vi "FPGAController_v4.vi"() -> ()   [LabVIEW 2013]
uses:
  <vilib>/Utility/miscctls.llb/LVPointTypeDef.ctl
  <userlib>/_OpenG.lib/file/file.llb/Strip Path Extension - Path__ogtk.vi
  <userlib>/_OpenG.lib/comparison/comparison.llb/Boolean Changed__ogtk.vi
  <vilib>/FPGAPlugInAG/PXI-7954R/niLvFpga_Open_PXI-7954R.vi
  <vilib>/addons/database/Connection.llb/Conn Execute.vi
  <vilib>/addons/database/Recordset.llb/Rec Fetch Recordset Data (R).vi
  <vilib>/addons/database/Recordset.llb/Rec Destroy - Connection.vi
  <vilib>/Utility/error.llb/Error Cluster From Error Code.vi
  <vilib>/rvi/errors/niLvFpgaAdjustHostInterfaceError.vi
  <vilib>/FPGAPlugInAG/PXI-7954R/niLvFpga_Close_PXI-7954R.vi
  <vilib>/rvi/interface/nirviOpenFPGA/nirviOpenFPGA.xnode
  FPGA Bitfiles/correlationwithf_FPGATarget_FPGAcode60214_dpdmgs7o1BA.lvbitx
  <vilib>/rvi/interface/nirviMethod/nirviMethod.xnode
  <vilib>/FPGA/interface/niFpgaViExecutionMode.ctl
  <vilib>/rvi/interface/nirviReadWriteControl/nirviReadWriteControl.xnode
  <vilib>/addons/database/_DB Variant To Data/Database Variant To Data.xnode
  <vilib>/rvi/interface/nirviCloseFPGA/nirviCloseFPGA.xnode
  <vilib>/addons/database/NI_Database_API.lvlib
  NiFpgaLv.dll
panel:
  in  "Lower Threshold":bool
  in  "Raise Threshold":bool
  out "Update Threshold":bool
  in  "Min. Time\nBetween Shots (s)":dbl
  in  "Rate Limiting":bool
  out "Armed":bool
  in  "Use Delay?":bool
  in  "Add Delay":bool
  in  "Delay Name":string
  in  "Delay Value":dbl=3.0
  in  "Delay Ring":dbl(ring)=3.15039 items=["Ablation Chamber"=6.45, "LEIL Chamber"=4.318, "Thid Detector"=3.15039, "Custom"=0.0]
  in  "Rearm Trigger":bool
  in  "One Shot Mode":bool
  out "Last Update:":timestamp
  out "Updating FPGA":bool
  out "Sensitivity":dbl
  out "error out":errorcluster
  out "Low Mass Limit":fxp<+,31,17>
  out "High Mass Limit":fxp<+,31,17>
  out "stopping":bool
  in  "Auto Threshold":bool
  out "Peletron (MV)":dbl=2.0
  out "High Mass (kg)":dbl=inf
  out "Low Mass (kg)":dbl
  out "High Charge Limit":i16
  out "Low Charge Limit":i16
  out "High velocity count":i32=210
  out "Low velocity count":i32=21000
  in  "stop":bool
  in  "Peak-Threshold Factor":dbl=2.0
  out "Low Charge Limit (fC)":dbl
  out "High Charge Limit (fC)":dbl=100.0
  out "High Velocity":dbl=100000.0
  out "Low Velocity":dbl=1000.0
  out "Filter 7 Peak":i32=7483
  out "Filter 6 Peak":i32=9863
  out "Filter 5 Peak":i32=13910
  out "Filter 4 Peak":i32=18191
  out "Filter 3 Peak":i32=46254
  out "Filter 2 Peak":i32=120664
  out "Filter 1 Peak":i32=295996
  in  "Filter7 Threshold":i32=-21165
  in  "Filter6 Threshold":i32=-29358
  in  "Filter5 Threshold":i32=-41730
  in  "Filter4 Threshold":i32=-54306
  in  "Filter3 Threshold":i32=-138762
  in  "Filter2 Threshold":i32=-361992
  in  "Filter1 Threshold":i32=-887988
  in  "Zero Peak Values":bool
  in  "Assign Threshold":bool
  in  "Run Mode":bool
  # "Settings"
  # "Dubugging"
  # "Independent Variable"
  # "Low Vel."
  # "High Vel."
  # "Low Q (fC)"
  # "High Q (fC)"
  # "Plate Control While Loop Counter"
  # "Low Mass (kg)"
  # "High Mass (kg)"
  # "Sens. (V/pC)"
  # "Peletron (MV)"
  # "Current Value of Running Average"
  # "Peak Threshold Factor"
  # "Delay Trigger"
  # "Dist. from 2nd Det. (m)"
  # "Name"
  # "Peak Values"
  # "Peak 1"
  # "Peak 2"
  # "Peak 3"
  # "Peak 4"
  # "Peak 5"
  # "Peak 6"
  # "Peak 7"
  # "Thresholds"
  # "Threshold 1"
  # "Threshold 2"
  # "Threshold 3"
  # "Threshold 4"
  # "Threshold 5"
  # "Threshold 6"
  # "Threshold 7"
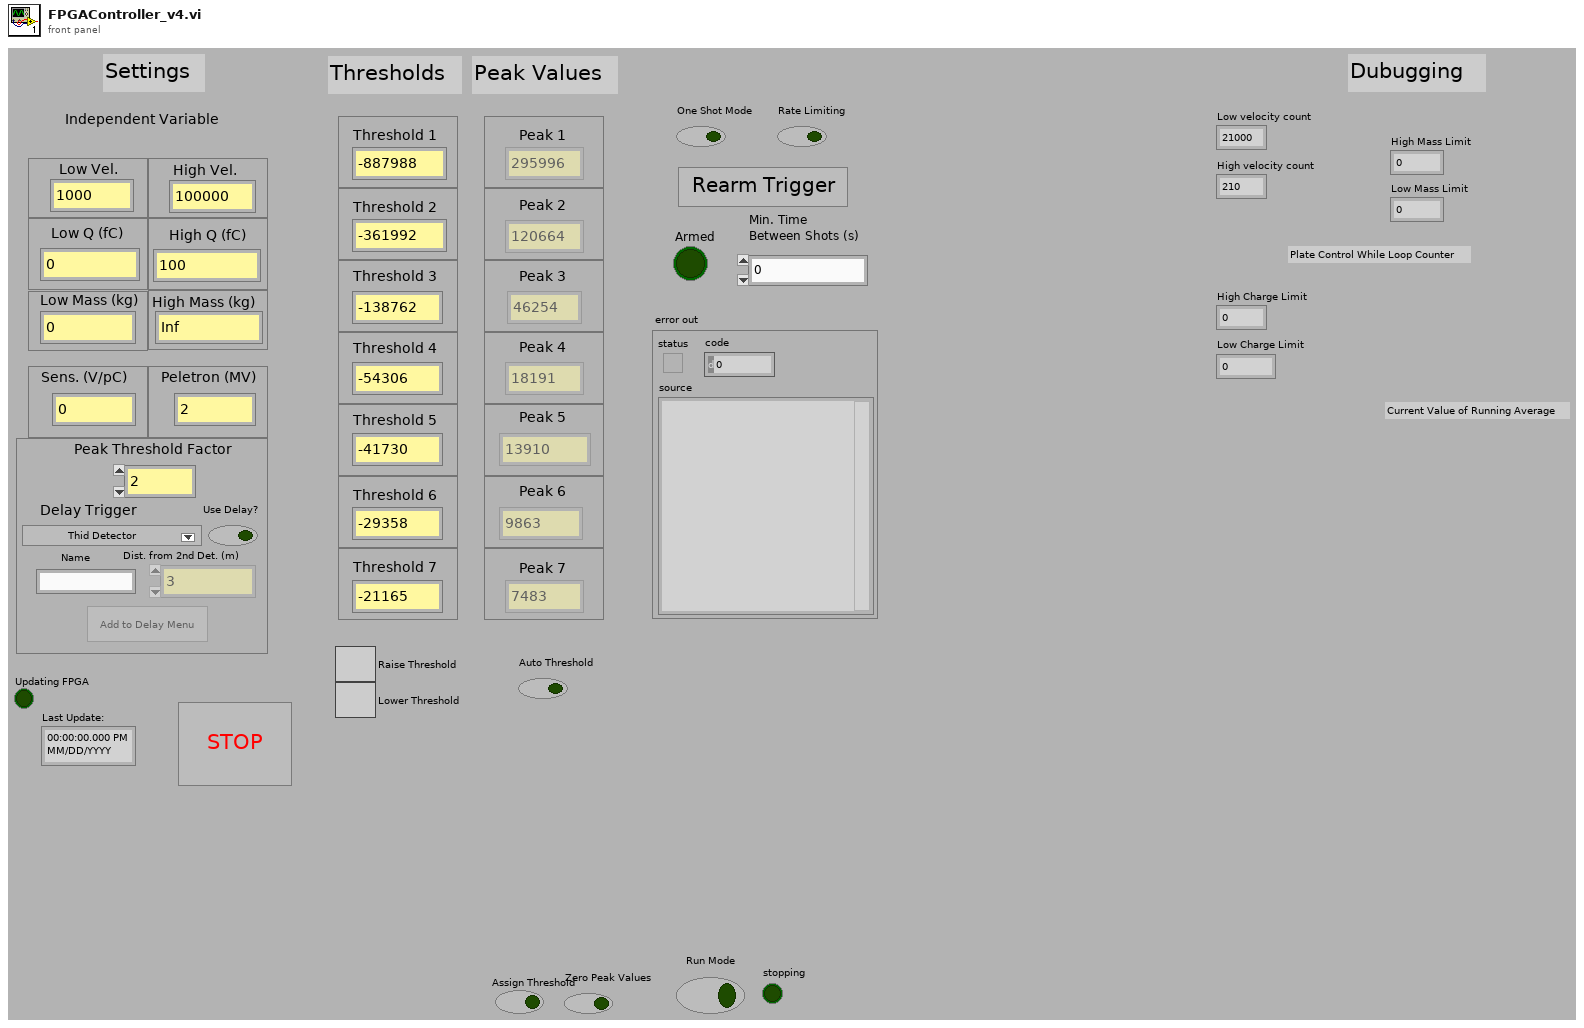
[diagram p1: front panel]
types:
  T1 = typedef "LVPointTypeDef.ctl" = cluster{"Horizontal":i16, "Vertical":i16}
  T2 = enum8{"Enabled", "Disabled", "Disabled and Grayed Out"}
  T3 = typedef "NI_Database_API.lvlib/Conn ObjectReference.ctl" = refnum<k1>
  T4 = cluster{"Filter 1 Peak":i32, "Filter 2 Peak":i32, "Filter 3 Peak":i32, "Filter 4 Peak":i32, "Filter 5 Peak":i32, "Filter 6 Peak":i32, "Filter 7 Peak":i32}
  T5 = typedef "NI_Database_API.lvlib/Rec ObjectReference.ctl" = refnum<k1>
  T6 = typedef "LVStringsAndValuesArrayTypeDef_DBL.ctl" = cluster{"String":string, "Value":dbl}[]
  T7 = cluster{"Numeric":dbl, "Numeric":dbl, "Numeric":dbl, "Numeric":dbl, "Numeric":dbl, "Numeric":dbl, dbl, dbl, "Value":dbl, fxp<+,16,7>, "Use Delay?":bool}
  T8 = cluster{"Low Velocity Count":i32, "High Velocity Count":i32, "Low Charge Limit (ADC ticks)":i16, "High Charge Limit (ADC ticks)":i16, "Low Mass (ADC*cycle^2)":i64, "High Mass (ADC*cycle^2)":i64, "Mult":fxp<+,16,7>, "Mult Use?":bool}
  T9 = cluster{"Filter 1 Detector 3 Correlation":i32, "Filter 2 Detector 3 Correlation":i32, "Filter 3 Detector 3 Correlation":i32, "Filter 4 Detector 3 Correlation":i32, "Filter 5 Detector 3 Correlation":i32, "Filter 6 Detector 3 Correlation":i32, "Filter 7 Detector 3 Correlation":i32}
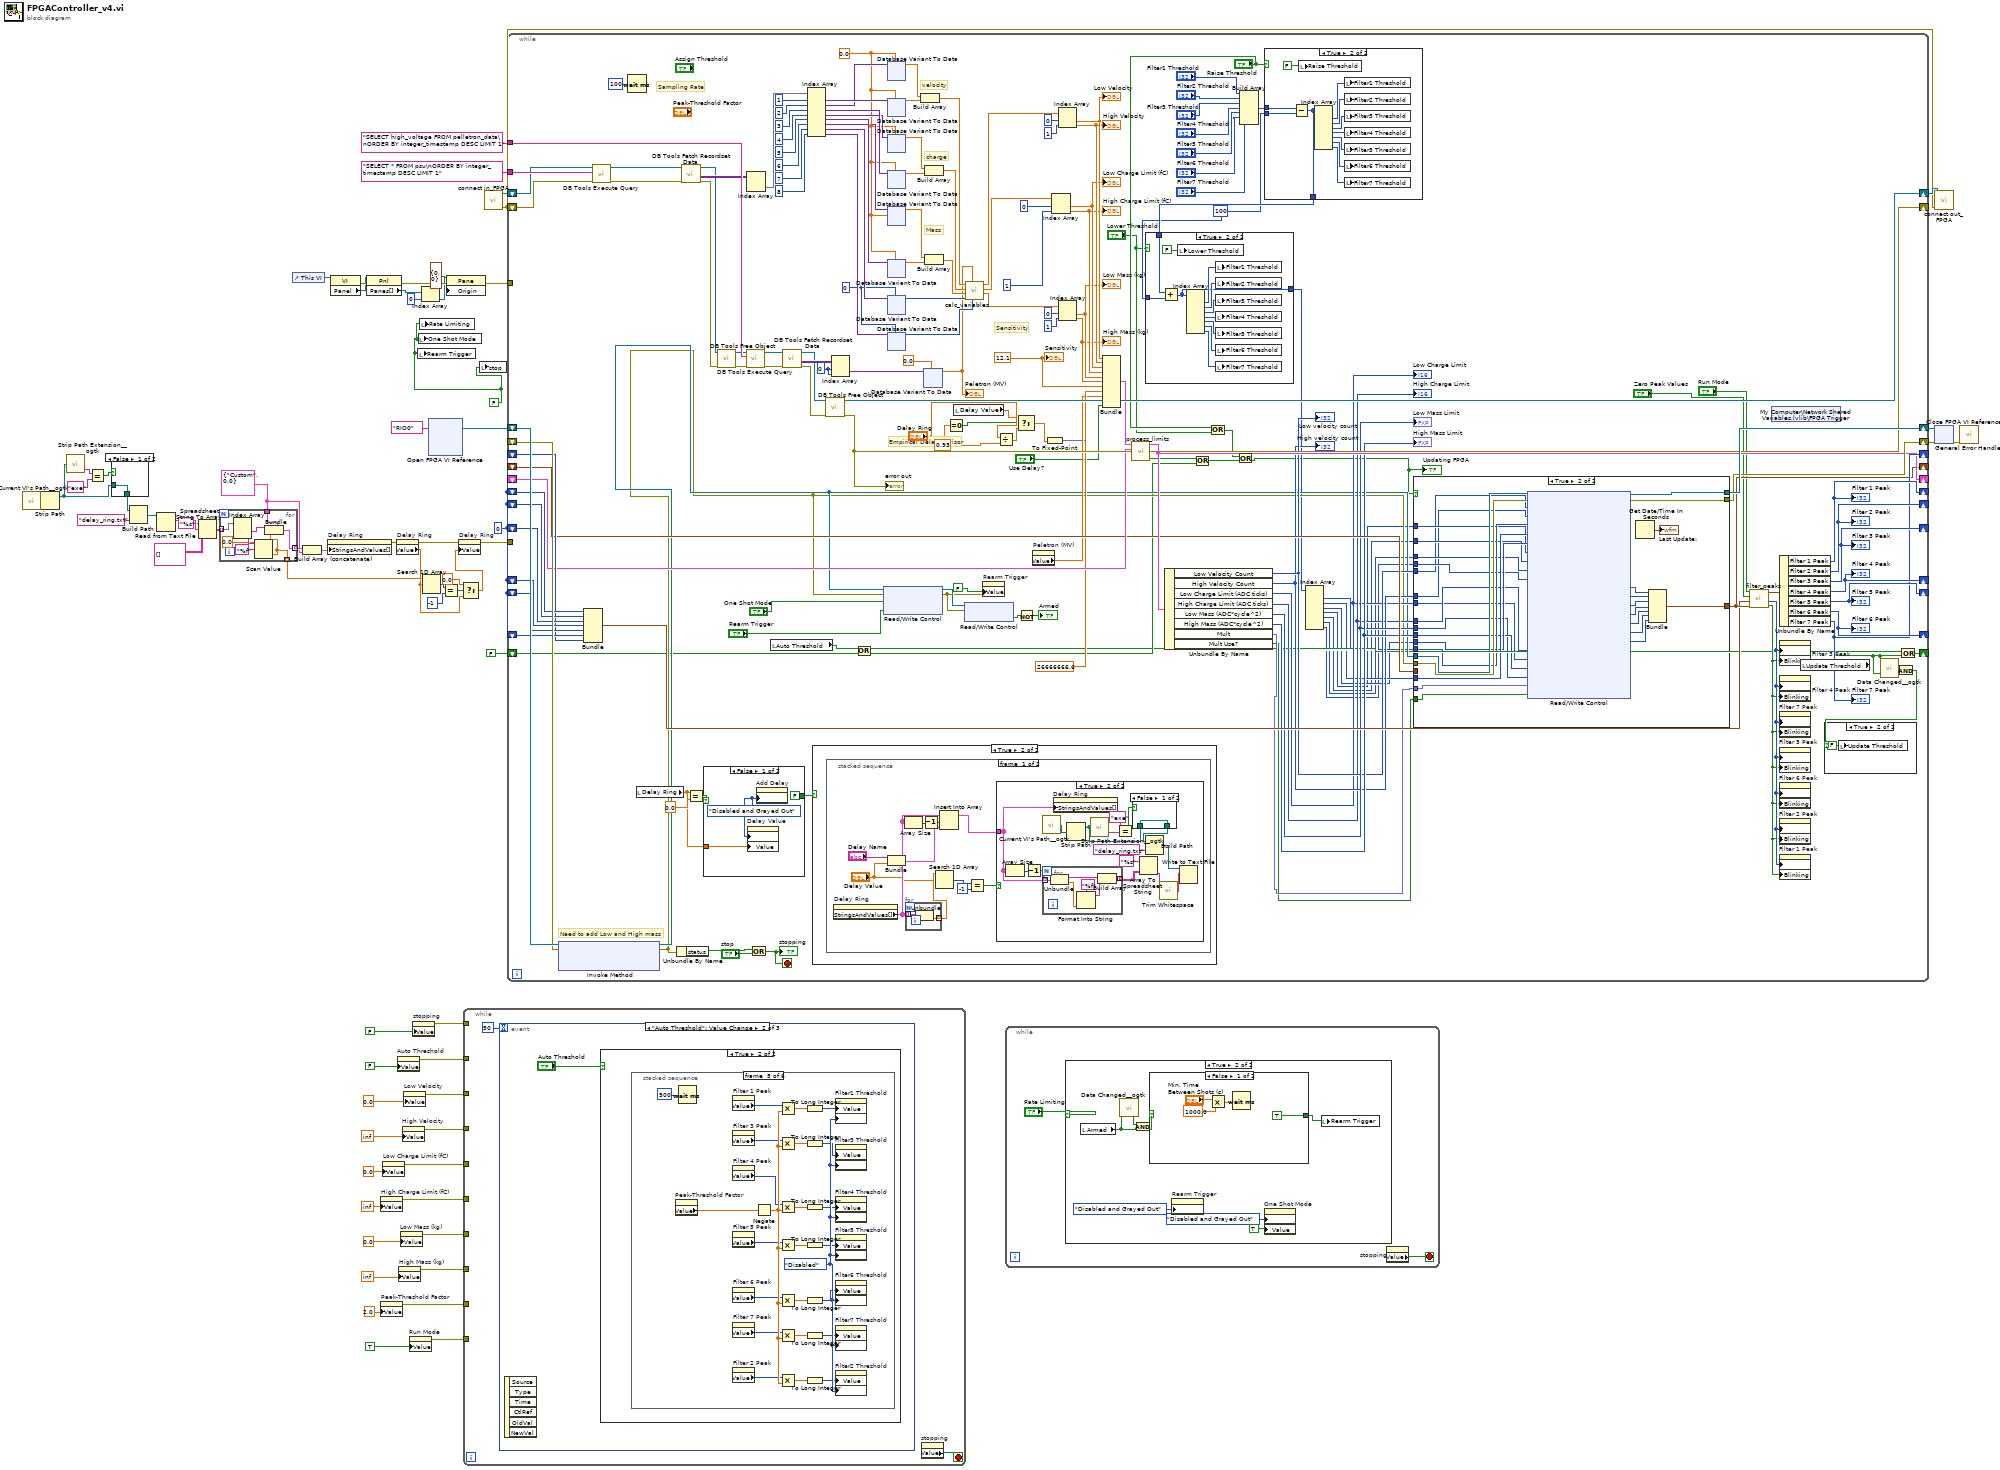
[diagram p0: block diagram]
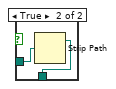
[diagram p2: hidden frame]
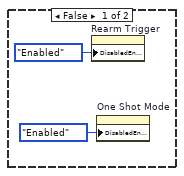
[diagram p3: hidden frame]
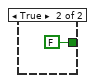
[diagram p4: hidden frame]
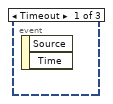
[diagram p5: hidden frame]
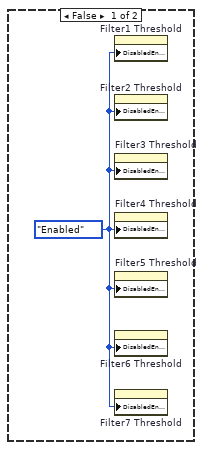
[diagram p6: hidden frame]
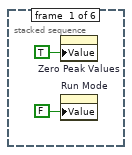
[diagram p7: hidden frame]
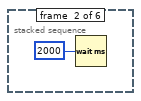
[diagram p8: hidden frame]
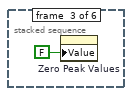
[diagram p9: hidden frame]
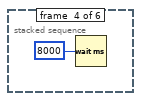
[diagram p10: hidden frame]
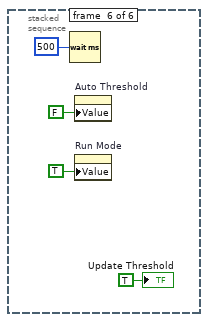
[diagram p11: hidden frame]
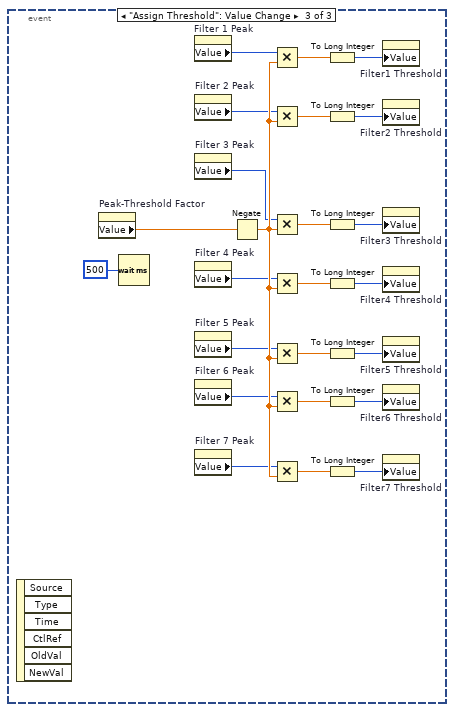
[diagram p12: hidden frame]
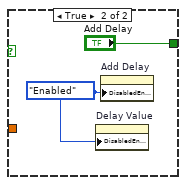
[diagram p16: hidden frame]
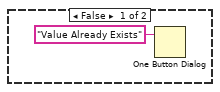
[diagram p18: hidden frame]
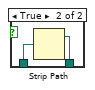
[diagram p19: hidden frame]
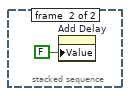
[diagram p20: hidden frame]
diagram:
  w17 = cluster{"String":string, "Value":dbl} {"String"="Custom", "Value"=0.0}
  w27 = FALSE
  w66 = 0
  n1 = call <userlib>:"Current VI's Path__ogtk.vi"() -> ("Current VI's Path (+ Relative)"=w26:path)  [unwired: 1 in]
  n2 = Strip Path(path=w26) -> (stripped path=w12:path)  [unwired: 1 out]
  n3 = call-poly <userlib>:"Strip Path Extension__ogtk.vi"("path"=w12) -> ("extension"=w16:string)  [unwired: 1 out]
  n4 = Equal?(x=w16, y="exe") -> (x = y?=w13:bool)
  n5 = case shown="False" w13 {
    tunnel: w12 -> [w68 w70]
    tunnel: [w68 w69] -> w11
    frame False {
    }
    frame True {
      n6 = Strip Path(path=w70) -> (stripped path=w69:path)  [unwired: 1 out]
    }
  }
  n7 = Build Path(base path=w11, name or relative path="delay_ring.txt") -> (appended path=w14:path)
  n8 = Read from Text File(file (use dialog)=w14) -> (text=w24:string)  [unwired: 3 in, 3 out]
  n9 = Spreadsheet String To Array(format string="%s", spreadsheet string=w24, array type (2D Dbl)=string[][] []) -> (array=w21:string[][])  [unwired: 1 in]
  n10 = for {
    tunnel: w21 -> [w78] mode=indexing
    tunnel: w17 -> [w76]
    tunnel: [w72] -> w18 mode=indexing
    tunnel: [w71] -> w10 mode=indexing
    n11 = Index Array(array=w78) -> (element #1=w77:string, element #2=w75:string)  [unwired: 2 in]
    n12 = Scan Value(string=w75, format string="%f", default (0 dbl)=0.0) -> (value=w71:dbl)  [unwired: 1 out]
    n13 = Bundle(cluster=w76, "String"=w77, "Value"=w71) -> (w72:cluster{"String":string, "Value":dbl})
  }
  n14 = control-ref of="This VI"() -> (w38:refnum<vi>)
  n15 = Build Array (concatenate)(w18, w17) -> (w20:cluster{"String":string, "Value":dbl}[])
  n16 = property on="Delay Ring" class="Ring (strict)"("StringsAndValues[]"=w20) -> (error out=w19:errorcluster)  [unwired: 2 in, 1 out]
  n17 = property class="VI"(reference=w38) -> (error out=w37:errorcluster, "Panel"=w36:refnum<vi>)  [unwired: 1 in, 1 out]
  n18 = property class="Pnl"(reference=w36, error in=w37) -> (error out=w35:errorcluster, "Panes[]"=w34:refnum<vi>[])  [unwired: 1 out]
  n19 = property on="High Charge Limit (fC)" class="DigNum (strict)"("Value"=inf ("High Charge Limit (fC)")) -> (error out=w53:errorcluster)  [unwired: 2 in, 1 out]
  n20 = property on="Peak-Threshold Factor" class="DigNum (strict)"("Value"=2.0 ("Peak-Threshold Factor")) -> (error out=w47:errorcluster)  [unwired: 2 in, 1 out]
  n21 = property on="Low Charge Limit (fC)" class="DigNum (strict)"("Value"=0.0 ("Low Charge Limit (fC)")) -> (error out=w55:errorcluster)  [unwired: 2 in, 1 out]
  n22 = property on="Delay Ring" class="Ring (strict)"(error in=w19) -> (error out=w9:errorcluster, "Value"=w3:dbl)  [unwired: 1 in, 1 out]
  n23 = property on="Auto Threshold" class="Bool (strict)"("Value"=FALSE ("Auto Threshold")) -> (error out=w61:errorcluster)  [unwired: 2 in, 1 out]
  n24 = property on="High Mass (kg)" class="DigNum (strict)"("Value"=inf ("High Mass (kg)")) -> (error out=w49:errorcluster)  [unwired: 2 in, 1 out]
  n25 = property on="Low Mass (kg)" class="DigNum (strict)"("Value"=0.0 ("Low Mass (kg)")) -> (error out=w51:errorcluster)  [unwired: 2 in, 1 out]
  n26 = property on="High Velocity" class="DigNum (strict)"("Value"=inf ("High Velocity")) -> (error out=w57:errorcluster)  [unwired: 2 in, 1 out]
  n27 = property on="Low Velocity" class="DigNum (strict)"("Value"=0.0 ("Low Velocity")) -> (error out=w59:errorcluster)  [unwired: 2 in, 1 out]
  n28 = property on="Run Mode" class="Bool (strict)"("Value"=TRUE ("Run Mode")) -> (error out=w45:errorcluster)  [unwired: 2 in, 1 out]
  n29 = property on="stopping" class="Bool (strict)"("Value"=FALSE ("stopping")) -> (error out=w63:errorcluster)  [unwired: 2 in, 1 out]
  n30 = local write "Rearm Trigger"(w27) -> ()
  n31 = local write "One Shot Mode"(w27) -> ()
  n32 = local write "Rate Limiting"(w27) -> ()
  n33 = Index Array(array=w34, index=0) -> (element=w32:refnum<vi>)
  n34 = Search 1D Array(1D array=w10, element=w3) -> (index of element=w7:i32)  [unwired: 1 in]
  n35 = xnode "Open FPGA VI Reference"("resource name"=tag "RIO0") -> ("FPGA VI Reference Out"=w29:refnum<k20>)  [unwired: 1 in, 1 out]
  n36 = Equal?(x=w7, y=-1) -> (x = y?=w5:bool)
  n37 = property class="Pane"(reference=w32, error in=w35, "Origin"=T1 {"Horizontal"=0, "Vertical"=0}) -> (error out=w30:errorcluster)  [unwired: 1 out]
  n38 = Select(t=0.0, s=w5, f=w3) -> (s? t:f=w4:dbl)
  n39 = property on="Delay Ring" class="Ring (strict)"(error in=w9, "Value"=w4) -> (error out=w8:errorcluster)  [unwired: 1 in, 1 out]
  n40 = while {
    tunnel: w63 -> [_]
    tunnel: w61 -> [_]
    tunnel: w59 -> [_]
    tunnel: w57 -> [_]
    tunnel: w55 -> [_]
    tunnel: w53 -> [_]
    tunnel: w51 -> [_]
    tunnel: w49 -> [_]
    tunnel: w47 -> [_]
    tunnel: w45 -> [_]
    stop <- w80 stop-if-true
    n41 = event shown="[1] \"Auto Threshold\": Value Change" {
      selector: _ -> [_ _ _]
      dyn-events: _ -> [_ _ _]
      timeout: 50 -> [_ _ _]
      event Timeout {
        n42 = event-data() -> ()  [unwired: 1 in, 2 out]
      }
      event "Auto Threshold": Value Change {
        n43 = event-data() -> ()  [unwired: 1 in, 6 out]
        n44 = case shown="True" "Auto Threshold" {
          frame False {
            w82 = T2."Enabled" ("Disabled")
            n45 = property on="Filter1 Threshold" class="DigNum (strict)"("DisabledEnum"=w82) -> ()  [unwired: 2 in, 2 out]
            n46 = property on="Filter2 Threshold" class="DigNum (strict)"("DisabledEnum"=w82) -> ()  [unwired: 2 in, 2 out]
            n47 = property on="Filter3 Threshold" class="DigNum (strict)"("DisabledEnum"=w82) -> ()  [unwired: 2 in, 2 out]
            n48 = property on="Filter4 Threshold" class="DigNum (strict)"("DisabledEnum"=w82) -> ()  [unwired: 2 in, 2 out]
            n49 = property on="Filter5 Threshold" class="DigNum (strict)"("DisabledEnum"=w82) -> ()  [unwired: 2 in, 2 out]
            n50 = property on="Filter6 Threshold" class="DigNum (strict)"("DisabledEnum"=w82) -> ()  [unwired: 2 in, 2 out]
            n51 = property on="Filter7 Threshold" class="DigNum (strict)"("DisabledEnum"=w82) -> ()  [unwired: 2 in, 2 out]
          }
          frame True {
            n52 = stacked-sequence {
              frame #0 {
                n53 = property on="Zero Peak Values" class="Bool (strict)"("Value"=TRUE ("Zero Peak Values")) -> ()  [unwired: 2 in, 2 out]
                n54 = property on="Run Mode" class="Bool (strict)"("Value"=FALSE ("Run Mode")) -> ()  [unwired: 2 in, 2 out]
              }
              frame #1 {
                n55 = Wait (ms)(milliseconds to wait=u32 2000) -> ()  [unwired: 1 out]
              }
              frame #2 {
                n56 = property on="Zero Peak Values" class="Bool (strict)"("Value"=FALSE ("Zero Peak Values")) -> ()  [unwired: 2 in, 2 out]
              }
              frame #3 {
                n57 = Wait (ms)(milliseconds to wait=u32 8000) -> ()  [unwired: 1 out]
              }
              frame #4 {
                w112 = T2."Disabled" ("Disabled")
                n58 = property on="Peak-Threshold Factor" class="DigNum (strict)"() -> ("Value"=w97:dbl)  [unwired: 2 in, 2 out]
                n59 = Wait (ms)(milliseconds to wait=u32 500) -> ()  [unwired: 1 out]
                n60 = property on="Filter 1 Peak" class="DigNum (strict)"() -> ("Value"=w95:i32)  [unwired: 2 in, 2 out]
                n61 = property on="Filter 3 Peak" class="DigNum (strict)"() -> ("Value"=w93:i32)  [unwired: 2 in, 2 out]
                n62 = property on="Filter 4 Peak" class="DigNum (strict)"() -> ("Value"=w92:i32)  [unwired: 2 in, 2 out]
                n63 = property on="Filter 5 Peak" class="DigNum (strict)"() -> ("Value"=w91:i32)  [unwired: 2 in, 2 out]
                n64 = property on="Filter 6 Peak" class="DigNum (strict)"() -> ("Value"=w90:i32)  [unwired: 2 in, 2 out]
                n65 = property on="Filter 7 Peak" class="DigNum (strict)"() -> ("Value"=w89:i32)  [unwired: 2 in, 2 out]
                n66 = property on="Filter 2 Peak" class="DigNum (strict)"() -> ("Value"=w94:i32)  [unwired: 2 in, 2 out]
                n67 = Negate(x=w97) -> (-x=w96:dbl)
                n68 = Multiply(x=w95, y=w96) -> (x*y=w111:dbl)
                n69 = Multiply(x=w93, y=w96) -> (x*y=w107:dbl)
                n70 = Multiply(x=w92, y=w96) -> (x*y=w105:dbl)
                n71 = Multiply(x=w91, y=w96) -> (x*y=w103:dbl)
                n72 = Multiply(x=w90, y=w96) -> (x*y=w101:dbl)
                n73 = Multiply(x=w89, y=w96) -> (x*y=w99:dbl)
                n74 = Multiply(x=w94, y=w96) -> (x*y=w109:dbl)
                n75 = To Long Integer(number=w111) -> (32bit integer=w110:i32)
                n76 = To Long Integer(number=w107) -> (32bit integer=w106:i32)
                n77 = To Long Integer(number=w105) -> (32bit integer=w104:i32)
                n78 = To Long Integer(number=w103) -> (32bit integer=w102:i32)
                n79 = To Long Integer(number=w101) -> (32bit integer=w100:i32)
                n80 = To Long Integer(number=w99) -> (32bit integer=w98:i32)
                n81 = To Long Integer(number=w109) -> (32bit integer=w108:i32)
                n82 = property on="Filter1 Threshold" class="DigNum (strict)"("Value"=w110, "DisabledEnum"=w112) -> ()  [unwired: 2 in, 2 out]
                n83 = property on="Filter3 Threshold" class="DigNum (strict)"("Value"=w106, "DisabledEnum"=w112) -> ()  [unwired: 2 in, 2 out]
                n84 = property on="Filter4 Threshold" class="DigNum (strict)"("Value"=w104, "DisabledEnum"=w112) -> ()  [unwired: 2 in, 2 out]
                n85 = property on="Filter5 Threshold" class="DigNum (strict)"("Value"=w102, "DisabledEnum"=w112) -> ()  [unwired: 2 in, 2 out]
                n86 = property on="Filter6 Threshold" class="DigNum (strict)"("Value"=w100, "DisabledEnum"=w112) -> ()  [unwired: 2 in, 2 out]
                n87 = property on="Filter7 Threshold" class="DigNum (strict)"("Value"=w98, "DisabledEnum"=w112) -> ()  [unwired: 2 in, 2 out]
                n88 = property on="Filter2 Threshold" class="DigNum (strict)"("Value"=w108, "DisabledEnum"=w112) -> ()  [unwired: 2 in, 2 out]
              }
              frame #5 {
                n89 = Wait (ms)(milliseconds to wait=u32 500) -> ()  [unwired: 1 out]
                n90 = property on="Auto Threshold" class="Bool (strict)"("Value"=FALSE ("Auto Threshold")) -> ()  [unwired: 2 in, 2 out]
                n91 = property on="Run Mode" class="Bool (strict)"("Value"=TRUE ("Run Mode")) -> ()  [unwired: 2 in, 2 out]
                "Update Threshold" <- TRUE ("Update Threshold")
              }
            }
          }
        }
      }
      event "Assign Threshold": Value Change {
        n92 = event-data() -> ()  [unwired: 1 in, 6 out]
        n93 = property on="Peak-Threshold Factor" class="DigNum (strict)"() -> ("Value"=w131:dbl)  [unwired: 2 in, 2 out]
        n94 = Wait (ms)(milliseconds to wait=u32 500) -> ()  [unwired: 1 out]
        n95 = property on="Filter 1 Peak" class="DigNum (strict)"() -> ("Value"=w130:i32)  [unwired: 2 in, 2 out]
        n96 = property on="Filter 2 Peak" class="DigNum (strict)"() -> ("Value"=w129:i32)  [unwired: 2 in, 2 out]
        n97 = property on="Filter 3 Peak" class="DigNum (strict)"() -> ("Value"=w128:i32)  [unwired: 2 in, 2 out]
        n98 = property on="Filter 4 Peak" class="DigNum (strict)"() -> ("Value"=w127:i32)  [unwired: 2 in, 2 out]
        n99 = property on="Filter 5 Peak" class="DigNum (strict)"() -> ("Value"=w126:i32)  [unwired: 2 in, 2 out]
        n100 = property on="Filter 6 Peak" class="DigNum (strict)"() -> ("Value"=w125:i32)  [unwired: 2 in, 2 out]
        n101 = property on="Filter 7 Peak" class="DigNum (strict)"() -> ("Value"=w124:i32)  [unwired: 2 in, 2 out]
        n102 = Negate(x=w131) -> (-x=w133:dbl)
        n103 = Multiply(x=w130, y=w133) -> (x*y=w140:dbl)
        n104 = Multiply(x=w129, y=w133) -> (x*y=w138:dbl)
        n105 = Multiply(x=w128, y=w133) -> (x*y=w137:dbl)
        n106 = Multiply(x=w127, y=w133) -> (x*y=w136:dbl)
        n107 = Multiply(x=w126, y=w133) -> (x*y=w135:dbl)
        n108 = Multiply(x=w125, y=w133) -> (x*y=w134:dbl)
        n109 = Multiply(x=w124, y=w133) -> (x*y=w139:dbl)
        n110 = To Long Integer(number=w140) -> (32bit integer=w123:i32)
        n111 = To Long Integer(number=w138) -> (32bit integer=w122:i32)
        n112 = To Long Integer(number=w137) -> (32bit integer=w121:i32)
        n113 = To Long Integer(number=w136) -> (32bit integer=w120:i32)
        n114 = To Long Integer(number=w135) -> (32bit integer=w119:i32)
        n115 = To Long Integer(number=w134) -> (32bit integer=w118:i32)
        n116 = To Long Integer(number=w139) -> (32bit integer=w117:i32)
        n117 = property on="Filter1 Threshold" class="DigNum (strict)"("Value"=w123) -> ()  [unwired: 2 in, 2 out]
        n118 = property on="Filter2 Threshold" class="DigNum (strict)"("Value"=w122) -> ()  [unwired: 2 in, 2 out]
        n119 = property on="Filter3 Threshold" class="DigNum (strict)"("Value"=w121) -> ()  [unwired: 2 in, 2 out]
        n120 = property on="Filter4 Threshold" class="DigNum (strict)"("Value"=w120) -> ()  [unwired: 2 in, 2 out]
        n121 = property on="Filter5 Threshold" class="DigNum (strict)"("Value"=w119) -> ()  [unwired: 2 in, 2 out]
        n122 = property on="Filter6 Threshold" class="DigNum (strict)"("Value"=w118) -> ()  [unwired: 2 in, 2 out]
        n123 = property on="Filter7 Threshold" class="DigNum (strict)"("Value"=w117) -> ()  [unwired: 2 in, 2 out]
      }
    }
    n124 = property on="stopping" class="Bool (strict)"() -> ("Value"=w80:bool)  [unwired: 2 in, 2 out]
  }
  n125 = local write "stop"(w27) -> ()
  n126 = call "connect in_FPGA.vi"() -> ("error out"=w39:errorcluster, "Database Connection"=w40:T3)  [unwired: 7 in, 1 out]
  n127 = while {
    shift-right: [w299] -> w65
    shift-left: w29 -> [w303]
    shift-right: [w298] -> w64
    shift-left: _ -> [w302]
    shift-right: [w294] -> _
    shift-left: w66 -> [w287]
    shift-right: [w293] -> _
    shift-left: w66 -> [w286]
    shift-right: [w292] -> _
    shift-left: w66 -> [w285]
    shift-right: [w291] -> _
    shift-left: w66 -> [w284]
    shift-right: [w290] -> _
    shift-left: w66 -> [w283]
    shift-right: [w296] -> _
    shift-left: w66 -> [w289]
    shift-right: [w295] -> _
    shift-left: w66 -> [w288]
    tunnel: "SELECT * FROM psu\nORDER BY integer_timestamp DESC LIMIT 1" ("SQL query") -> [w282]
    tunnel: "SELECT high_voltage FROM pelletron_data\nORDER BY integer_timestamp DESC LIMIT 1" ("SQL query") -> [w281]
    shift-right: [w277] -> w41
    shift-left: w40 -> [w280]
    shift-right: [w278] -> _
    shift-left: w39 -> [w279]
    shift-right: [w276] -> _
    shift-left: _ -> [w275]
    shift-right: [w273] -> _
    shift-left: _ -> [w274]
    tunnel: w30 -> [_]
    tunnel: w8 -> [_]
    shift-right: [w173] -> _
    shift-left: FALSE -> [w176]
    stop <- w297 stop-if-true
    w167 = 100
    w229 = 0 ("index (row)")
    w237 = i8 0
    w238 = 0.0
    w203 = 12.1
    # "charge"
    # "Empirical Delay Divisor"
    # "Mass"
    # "velocity"
    # "Sensitivity"
    # "Sampling Rate"
    # "Need to add Low and High mass"
    n128 = xnode "Invoke Method"("FPGA VI Reference In"=w303, "error in"=w302) -> ("FPGA VI Reference Out"=w196:refnum<k20>, "error out"=w195:errorcluster)  [unwired: 1 out]
    n129 = Bundle("Filter 1 Peak"=w289, "Filter 2 Peak"=w288, "Filter 3 Peak"=w287, "Filter 4 Peak"=w286, "Filter 5 Peak"=w285, "Filter 6 Peak"=w284, "Filter 7 Peak"=w283) -> (w269:T4)  [unwired: 1 in]
    n130 = call-poly <vilib>:"DB Tools Execute Query.vi"("error in (no error)"=w279, "SQL query"=w282, "connection reference"=w280) -> ("error out"=w257:errorcluster, "recordset reference"=w258:T5)  [unwired: 5 in]
    n131 = Wait (ms)(milliseconds to wait=u32 100) -> ()  [unwired: 1 out]
    n132 = local read "Delay Ring"() -> (w177:dbl)
    n133 = Unbundle By Name(w195) -> ("status"=w301:bool)
    n134 = call-poly <vilib>:"DB Tools Fetch Recordset Data.vi"("error in (no error)"=w257, "recordset reference"=w258) -> ("error out"=w235:errorcluster, "recordset data"=w248:variant[][], "recordset reference out"=w236:T5)  [unwired: 3 in]
    n135 = Equal?(x=w177, y=0.0) -> (x = y?=w178:bool)
    n136 = case shown="False" w178 {
      tunnel: [FALSE ("Add Delay") "Add Delay"] -> w200
      tunnel: w177 -> [w330 _]
      frame False {
        w331 = T2."Disabled and Grayed Out" ("Disabled")
        n137 = property on="Delay Value" class="DigNum (strict)"("DisabledEnum"=w331, "Value"=w330) -> ()  [unwired: 2 in, 2 out]
        n138 = property on="Add Delay" class="Bool (strict)"("DisabledEnum"=w331) -> ()  [unwired: 2 in, 2 out]
      }
      frame True {
        w332 = T2."Enabled" ("Disabled")
        n139 = property on="Delay Value" class="DigNum (strict)"("DisabledEnum"=w332) -> ()  [unwired: 2 in, 2 out]
        n140 = property on="Add Delay" class="Bool (strict)"("DisabledEnum"=w332) -> ()  [unwired: 2 in, 2 out]
      }
    }
    n141 = call-poly <vilib>:"DB Tools Free Object.vi"("error in (no error)"=w235, "recordset reference"=w236) -> ("error out"=w233:errorcluster, "connection reference"=w234:T3)  [unwired: 8 in]
    n142 = call-poly <vilib>:"DB Tools Execute Query.vi"("error in (no error)"=w233, "SQL query"=w281, "connection reference"=w234) -> ("error out"=w231:errorcluster, "recordset reference"=w232:T5)  [unwired: 5 in]
    n143 = Index Array(array=w248) -> (element=w247:variant[])  [unwired: 2 in]
    n144 = Or(x=w301, y="stop") -> (x .or. y?=w297:bool)
    "stopping" <- w297
    n145 = local read "Auto Threshold"() -> (w174:bool)
    n146 = call-poly <vilib>:"DB Tools Fetch Recordset Data.vi"("error in (no error)"=w231, "recordset reference"=w232) -> ("error out"=w204:errorcluster, "recordset data"=w230:variant[][], "recordset reference out"=w205:T5)  [unwired: 3 in]
    n147 = Index Array(array=w247, index #1=1 ("index"), index #2=2 ("index"), index #3=3 ("index"), index #4=4 ("index"), index #5=5 ("index"), index #6=6 ("index"), index #7=7 ("index"), index #8=8 ("index")) -> (element #1=w246:variant, element #2=w245:variant, element #3=w244:variant, element #4=w243:variant, element #5=w242:variant, element #6=w241:variant, element #7=w240:variant, element #8=w239:variant)
    n148 = case shown="True" w200 {
      frame False {
      }
      frame True {
        n149 = stacked-sequence {
          frame #0 {
            n150 = property on="Delay Ring" class="Ring (strict)"() -> ("StringsAndValues[]"=w336:T6)  [unwired: 2 in, 2 out]
            n151 = Bundle("Delay Name"="Delay Name", "Delay Value"="Delay Value") -> (w341:cluster{"Delay Name":string, "Delay Value":dbl})  [unwired: 1 in]
            n152 = Array Size(array=w336) -> (size(s)=w339:i32)
            n153 = for {
              tunnel: w336 -> [w346] mode=indexing
              tunnel: [w345] -> w335 mode=indexing
              n154 = Unbundle(w346) -> ("Value"=w345:dbl)  [unwired: 1 out]
            }
            n155 = Decrement(x=w339) -> (x-1=w338:i32)
            n156 = Search 1D Array(1D array=w335, element="Delay Value") -> (index of element=w343:i32)  [unwired: 1 in]
            n157 = Insert Into Array(array=w336, index=w338, new element=w341) -> (w340:T6)
            n158 = Equal?(x=w343, y=-1) -> (x = y?=w337:bool)
            n159 = case shown="True" w337 {
              tunnel: w340 -> [_ w355]
              frame False {
                n160 = One Button Dialog(message="Value Already Exists") -> ()  [unwired: 1 in, 1 out]
              }
              frame True {
                n161 = Array Size(array=w355) -> (size(s)=w357:i32)
                n162 = Decrement(x=w357) -> (x-1=w356:i32)
                n163 = call <userlib>:"Current VI's Path__ogtk.vi"() -> ("Current VI's Path (+ Relative)"=w361:path)  [unwired: 1 in]
                n164 = for {
                  N: w356 -> [_]
                  tunnel: w355 -> [w371] mode=indexing
                  tunnel: [w366] -> w358 mode=indexing
                  n165 = Unbundle(w371) -> ("String"=w367:string, "Value"=w370:dbl)
                  n166 = Format Into String(format string="%f", w370) -> (resulting string=w368:string)  [unwired: 2 in, 1 out]
                  n167 = Build Array(w367, w368) -> (w366:string[])
                }
                n168 = property on="Delay Ring" class="Ring (strict)"("StringsAndValues[]"=w355) -> ()  [unwired: 2 in, 2 out]
                n169 = Strip Path(path=w361) -> (stripped path=w349:path)  [unwired: 1 out]
                n170 = call-poly <userlib>:"Strip Path Extension__ogtk.vi"("path"=w349) -> ("extension"=w352:string)  [unwired: 1 out]
                n171 = Equal?(x="exe", y=w352) -> (x = y?=w350:bool)
                n172 = case shown="False" w350 {
                  tunnel: w349 -> [w363 w365]
                  tunnel: [w363 w364] -> w348
                  frame False {
                  }
                  frame True {
                    n173 = Strip Path(path=w365) -> (stripped path=w364:path)  [unwired: 1 out]
                  }
                }
                n174 = Array To Spreadsheet String(array=w358, 3:"%s" ("format string")) -> (spreadsheet string=w354:string)  [unwired: 1 in]
                n175 = Build Path(base path=w348, name or relative path="delay_ring.txt") -> (appended path=w359:path)
                n176 = call <vilib>:"Trim Whitespace.vi"("string"=w354) -> ("trimmed string"=w353:string)  [unwired: 1 in]
                n177 = Write to Text File(file (use dialog)=w359, text=w353) -> ()  [unwired: 2 in, 3 out]
              }
            }
          }
          frame #1 {
            n178 = property on="Add Delay" class="Bool (strict)"("Value"=FALSE ("Add Delay")) -> ()  [unwired: 2 in, 2 out]
          }
        }
      }
    }
    n179 = call-poly <vilib>:"DB Tools Free Object.vi"("error in (no error)"=w204, "recordset reference"=w205) -> ("error out"=w278:errorcluster, "connection reference"=w277:T3)  [unwired: 8 in]
    "error out" <- w278
    n180 = Index Array(array=w230, index (row)=w229, index (col)=w229) -> (element=w228:variant)
    n181 = Or(x=w174, y=w176) -> (x .or. y?=w175:bool)
    n182 = xnode "Read/Write Control"("FPGA VI Reference In"=w196, "error in"=w195, "One Shot"="One Shot Mode", "Reset One Shot"="Rearm Trigger") -> ("FPGA VI Reference Out"=w189:refnum<k20>, "error out"=w188:errorcluster)
    n183 = xnode "Database Variant To Data"("database variant"=w245, "type"=w238) -> ("data"=w146:dbl)  [unwired: 1 in, 1 out]
    n184 = xnode "Database Variant To Data"("database variant"=w246, "type"=w238) -> ("data"=w147:dbl)  [unwired: 1 in, 1 out]
    n185 = xnode "Database Variant To Data"("database variant"=w243, "type"=w238) -> ("data"=w145:dbl)  [unwired: 1 in, 1 out]
    n186 = xnode "Database Variant To Data"("database variant"=w244, "type"=w238) -> ("data"=w144:dbl)  [unwired: 1 in, 1 out]
    n187 = xnode "Database Variant To Data"("database variant"=w241, "type"=w238) -> ("data"=w143:dbl)  [unwired: 1 in, 1 out]
    n188 = xnode "Database Variant To Data"("database variant"=w242, "type"=w238) -> ("data"=w142:dbl)  [unwired: 1 in, 1 out]
    n189 = xnode "Database Variant To Data"("database variant"=w240, "type"=w237) -> ("data"=w222:i8)  [unwired: 1 in, 1 out]
    n190 = xnode "Database Variant To Data"("database variant"=w239, "type"=w237) -> ("data"=w221:i8)  [unwired: 1 in, 1 out]
    n191 = Build Array(w146, w147) -> (w225:dbl[])
    n192 = xnode "Database Variant To Data"("database variant"=w228, "type"=0.0) -> ("data"=w141:dbl)  [unwired: 1 in, 1 out]
    "Peletron (MV)" <- w141
    n193 = Build Array(w145, w144) -> (w224:dbl[])
    n194 = Build Array(w143, w142) -> (w223:dbl[])
    n195 = Equal To 0?(x="Delay Ring") -> (x = 0?=w185:bool)
    n196 = local read "Delay Value"() -> (w182:dbl)
    n197 = xnode "Read/Write Control"("FPGA VI Reference In"=w189, "error in"=w188) -> ("Not Armed?"=w187:bool)  [unwired: 2 out]
    n198 = call "calc_variables.vi"("var2"=w221, "Peletron"=w141, "var1"=w222, "Mass"=w223, "Charge"=w224, "Velocity"=w225) -> ("Mass out"=w214:dbl[], "Charge out"=w217:dbl[], "Velocity out"=w220:dbl[])  [unwired: 3 in]
    n199 = property on="Rearm Trigger" class="Bool (strict)"(error in=w188, "Value"=FALSE ("Rearm Trigger")) -> ()  [unwired: 1 in, 2 out]
    n200 = Divide(x="Delay Ring", y=0.93) -> (x/y=w184:dbl)
    n201 = Select(t=w182, s=w185, f=w184) -> (s? t:f=w183:dbl)
    n202 = Not(x=w187) -> (.not. x?=→"Armed":bool)
    n203 = property on="Peletron (MV)" class="DigNum (strict)"() -> ("Value"=w226:dbl)  [unwired: 2 in, 2 out]
    n204 = To Fixed-Point(number=w183) -> (fixed-point=w199:fxp<+,16,7>)  [unwired: 1 in]
    n205 = Index Array(array=w217, index #1=0 ("index"), index #2=1 ("index")) -> (element #1=w209:dbl, element #2=w208:dbl)
    "High Charge Limit (fC)" <- w208
    "Low Charge Limit (fC)" <- w209
    n206 = Index Array(array=w220, index #1=0 ("index"), index #2=1 ("index")) -> (element #1=w211:dbl, element #2=w210:dbl)
    "High Velocity" <- w210
    "Low Velocity" <- w211
    n207 = Index Array(array=w214, index #1=0 ("index"), index #2=1 ("index")) -> (element #1=w207:dbl, element #2=w206:dbl)
    "Low Mass (kg)" <- w207
    "High Mass (kg)" <- w206
    n208 = Bundle("Numeric"=w211, "Numeric"=w210, "Numeric"=w209, "Numeric"=w208, "Numeric"=w207, "Numeric"=w206, w203, 26666666.6, "Value"=w226, w199, "Use Delay?"="Use Delay?") -> (w268:T7)  [unwired: 1 in]
    n209 = call "process_limits.vi"("old output cluster"=w275, "Input cluster"=w268) -> ("Update FPGA"=w202:bool, "output cluster"=w276:T8)  [unwired: 8 in]
    n210 = Unbundle By Name(w276) -> ("Low Velocity Count"=w264:i32, "High Velocity Count"=w263:i32, "Low Charge Limit (ADC ticks)"=w261:i16, "High Charge Limit (ADC ticks)"=w262:i16, "Low Mass (ADC*cycle^2)"=w266:i64, "High Mass (ADC*cycle^2)"=w267:i64, "Mult"=w198:fxp<+,16,7>, "Mult Use?"=w197:bool)
    "Low velocity count" <- w264
    "High velocity count" <- w263
    "High Charge Limit" <- w262
    "Low Charge Limit" <- w261
    "High Mass Limit" <- w267
    "Low Mass Limit" <- w266
    n211 = Or(x=w202, y=w175) -> (x .or. y?=w180:bool)
    n212 = Or(x="Raise Threshold", y="Lower Threshold") -> (x .or. y?=w148:bool)
    n213 = Or(x=w148, y=w180) -> (x .or. y?=w149:bool)
    "Updating FPGA" <- w149
    n214 = Build Array("Filter1 Threshold", "Filter2 Threshold", "Filter3 Threshold", "Filter4 Threshold", "Filter5 Threshold", "Filter6 Threshold", "Filter7 Threshold") -> (w169:i32[])
    n215 = case shown="True" "Raise Threshold" {
      tunnel: w169 -> [w316 w327]
      tunnel: [w316 w318] -> w168
      tunnel: w167 -> [_ w317]
      frame False {
      }
      frame True {
        n216 = Subtract(x=w327, y=w317) -> (x-y=w318:i32[])
        n217 = local write "Raise Threshold"(FALSE ("Raise Threshold")) -> ()
        n218 = Index Array(array=w318) -> (element #1=w325:i32, element #2=w324:i32, element #3=w323:i32, element #4=w322:i32, element #5=w321:i32, element #6=w320:i32, element #7=w319:i32)  [unwired: 7 in]
        n219 = local write "Filter1 Threshold"(w325) -> ()
        n220 = local write "Filter2 Threshold"(w324) -> ()
        n221 = local write "Filter3 Threshold"(w323) -> ()
        n222 = local write "Filter4 Threshold"(w322) -> ()
        n223 = local write "Filter5 Threshold"(w321) -> ()
        n224 = local write "Filter6 Threshold"(w320) -> ()
        n225 = local write "Filter7 Threshold"(w319) -> ()
      }
    }
    n226 = case shown="True" "Lower Threshold" {
      tunnel: w168 -> [w304 w315]
      tunnel: w167 -> [_ w314]
      tunnel: [w304 w305] -> w162
      frame False {
      }
      frame True {
        n227 = Add(x=w315, y=w314) -> (x+y=w305:i32[])
        n228 = local write "Lower Threshold"(FALSE ("Lower Threshold")) -> ()
        n229 = Index Array(array=w305) -> (element #1=w312:i32, element #2=w311:i32, element #3=w310:i32, element #4=w309:i32, element #5=w308:i32, element #6=w307:i32, element #7=w306:i32)  [unwired: 7 in]
        n230 = local write "Filter1 Threshold"(w312) -> ()
        n231 = local write "Filter2 Threshold"(w311) -> ()
        n232 = local write "Filter3 Threshold"(w310) -> ()
        n233 = local write "Filter4 Threshold"(w309) -> ()
        n234 = local write "Filter5 Threshold"(w308) -> ()
        n235 = local write "Filter6 Threshold"(w307) -> ()
        n236 = local write "Filter7 Threshold"(w306) -> ()
      }
    }
    n237 = Index Array(array=w162) -> (element #1=w165:i32, element #2=w163:i32, element #3=w160:i32, element #4=w158:i32, element #5=w156:i32, element #6=w154:i32, element #7=w152:i32)  [unwired: 7 in]
    n238 = case shown="True" w149 {
      tunnel: w196 -> [w374 w403]
      tunnel: w195 -> [w375 w402]
      tunnel: [w374 w401] -> w299
      tunnel: [w375 w400] -> w298
      tunnel: w165 -> [_ w399]
      tunnel: w163 -> [_ w398]
      tunnel: w160 -> [_ w397]
      tunnel: w158 -> [_ w396]
      tunnel: w156 -> [_ w395]
      tunnel: w154 -> [_ w394]
      tunnel: w152 -> [_ w393]
      tunnel: [w373 w379] -> w273
      tunnel: w267 -> [_ w385]
      tunnel: w266 -> [_ w384]
      tunnel: w264 -> [_ w383]
      tunnel: w263 -> [_ w382]
      tunnel: w262 -> [_ w381]
      tunnel: w261 -> [_ w380]
      tunnel: w274 -> [w373 _]
      tunnel: w198 -> [_ w377]
      tunnel: w197 -> [_ w376]
      frame False {
      }
      frame True {
        n239 = xnode "Read/Write Control"("FPGA VI Reference In"=w403, "error in"=w402, "Low Velocity Count"=w383, "High Velocity Count"=w382, "Filter 1 threshold"=w399, "Filter 2 threshold"=w398, "Filter 3 threshold"=w397, "Filter 4 threshold"=w396, "Filter 5 threshold"=w395, "Filter 6 threshold"=w394, "Filter 7 threshold"=w393, "High Charge Limit"=w381, "Low Charge Limit"=w380, "High Mass Limit"=w385, "Low Mass Limit"=w384, "Mult1"=w377, "Mult1 Use"=w376) -> ("FPGA VI Reference Out"=w401:refnum<k20>, "error out"=w400:errorcluster, "Filter 1 Detector 3 Correlation"=w392:i32, "Filter 2 Detector 3 Correlation"=w391:i32, "Filter 3 Detector 3 Correlation"=w390:i32, "Filter 4 Detector 3 Correlation"=w389:i32, "Filter 5 Detector 3 Correlation"=w388:i32, "Filter 6 Detector 3 Correlation"=w387:i32, "Filter 7 Detector 3 Correlation"=w386:i32)
        n240 = Get Date/Time In Seconds() -> (seconds since 1Jan1904=→"Last Update:":timestamp)
        n241 = Bundle("Filter 1 Detector 3 Correlation"=w392, "Filter 2 Detector 3 Correlation"=w391, "Filter 3 Detector 3 Correlation"=w390, "Filter 4 Detector 3 Correlation"=w389, "Filter 5 Detector 3 Correlation"=w388, "Filter 6 Detector 3 Correlation"=w387, "Filter 7 Detector 3 Correlation"=w386) -> (w379:T9)  [unwired: 1 in]
      }
    }
    n242 = call "filter_peaks.vi"("Correlation cluster"=w273, "Filter peak cluster"=w269, "Zero out"="Zero Peak Values", "Run Mode"="Run Mode") -> ("Blinking"=w260:bool, "status"=w265:T2, "Filter peak output"=w270:T4)  [unwired: 5 in]
    n243 = shared-variable "My Computer\\Network Shared Variables.lvlib\\FPGA Trigger"() -> ()  [unwired: 1 in, 2 out]
    n244 = Unbundle By Name(w270) -> ("Filter 1 Peak"=w296:i32, "Filter 2 Peak"=w295:i32, "Filter 3 Peak"=w294:i32, "Filter 4 Peak"=w293:i32, "Filter 5 Peak"=w292:i32, "Filter 6 Peak"=w291:i32, "Filter 7 Peak"=w290:i32)
    "Filter 1 Peak" <- w296
    "Filter 2 Peak" <- w295
    "Filter 3 Peak" <- w294
    "Filter 4 Peak" <- w293
    "Filter 5 Peak" <- w292
    "Filter 6 Peak" <- w291
    "Filter 7 Peak" <- w290
    n245 = property on="Filter 3 Peak" class="DigNum (strict)"("DisabledEnum"=w265, "Blinking"=w260) -> ()  [unwired: 2 in, 2 out]
    n246 = property on="Filter 4 Peak" class="DigNum (strict)"("DisabledEnum"=w265, "Blinking"=w260) -> ()  [unwired: 2 in, 2 out]
    n247 = property on="Filter 7 Peak" class="DigNum (strict)"("DisabledEnum"=w265, "Blinking"=w260) -> ()  [unwired: 2 in, 2 out]
    n248 = property on="Filter 5 Peak" class="DigNum (strict)"("DisabledEnum"=w265, "Blinking"=w260) -> ()  [unwired: 2 in, 2 out]
    n249 = property on="Filter 6 Peak" class="DigNum (strict)"("DisabledEnum"=w265, "Blinking"=w260) -> ()  [unwired: 2 in, 2 out]
    n250 = property on="Filter 2 Peak" class="DigNum (strict)"("DisabledEnum"=w265, "Blinking"=w260) -> ()  [unwired: 2 in, 2 out]
    n251 = property on="Filter 1 Peak" class="DigNum (strict)"("DisabledEnum"=w265, "Blinking"=w260) -> ()  [unwired: 2 in, 2 out]
    n252 = local read "Update Threshold"() -> (w171:bool)
    n253 = call-poly <userlib>:"Data Changed__ogtk.vi"("Boolean"=w171) -> ("Changed"=w172:bool)
    n254 = And(x=w172, y=w171) -> (x .and. y?=w170:bool)
    n255 = case shown="True" w170 {
      frame False {
      }
      frame True {
        n256 = local write "Update Threshold"(FALSE ("Update Threshold")) -> ()
      }
    }
    n257 = Or(x=w174, y=w171) -> (x .or. y?=w173:bool)
    "Sensitivity" <- w203
  }
  n258 = while {
    stop <- w693 stop-if-true
    n259 = case shown="True" "Rate Limiting" {
      frame False {
        n260 = property on="Rearm Trigger" class="Bool (strict)"("DisabledEnum"=T2."Enabled" ("Disabled")) -> ()  [unwired: 2 in, 2 out]
        n261 = property on="One Shot Mode" class="Bool (strict)"("DisabledEnum"=T2."Enabled" ("Disabled")) -> ()  [unwired: 2 in, 2 out]
      }
      frame True {
        n262 = local read "Armed"() -> (w698:bool)
        n263 = call-poly <userlib>:"Data Changed__ogtk.vi"("Boolean"=w698) -> ("Changed"=w696:bool)
        n264 = And(x=w696, y=w698) -> (x .and. y?=w697:bool)
        n265 = case shown="False" w697 {
          tunnel: [TRUE FALSE] -> w702
          frame False {
            n266 = Multiply(x="Min. Time\nBetween Shots (s)", y=1000.0) -> (x*y=w706:dbl)
            n267 = Wait (ms)(milliseconds to wait=w706) -> ()  [unwired: 1 out]
          }
          frame True {
          }
        }
        n268 = property on="Rearm Trigger" class="Bool (strict)"("DisabledEnum"=T2."Disabled and Grayed Out" ("Disabled")) -> ()  [unwired: 2 in, 2 out]
        n269 = property on="One Shot Mode" class="Bool (strict)"("DisabledEnum"=T2."Disabled and Grayed Out" ("Disabled"), "Value"=TRUE ("One Shot Mode")) -> ()  [unwired: 2 in, 2 out]
        n270 = local write "Rearm Trigger"(w702) -> ()
      }
    }
    n271 = property on="stopping" class="Bool (strict)"() -> ("Value"=w693:bool)  [unwired: 2 in, 2 out]
  }
  n272 = call "connect out_FPGA.vi"("error in (no error)"=w39, "connection reference"=w41) -> ()  [unwired: 9 in, 1 out]
  n273 = xnode "Close FPGA VI Reference"("FPGA VI Reference In"=w65, "error in"=w64) -> ("error out"=w67:errorcluster)
  n274 = call <vilib>:"General Error Handler.vi"("error in (no error)"=w67) -> ()  [unwired: 10 in, 5 out]
